vi "Measure DMM 3458A.vi"(8 "error in (no error)":errorcluster, 11 "VISA resource name":refnum<visa-resource-name>) -> (0 "error out":errorcluster, 3 "Display Value":sgl)   [LabVIEW 2016]
panel:
  out "Error Buffer":string
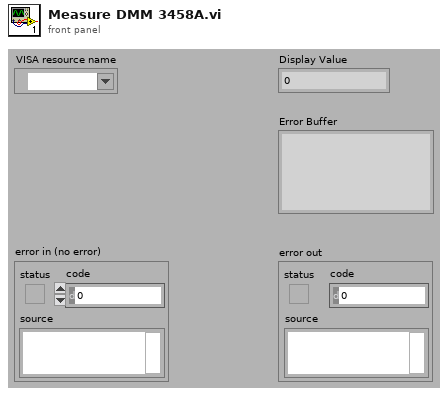
[diagram p1: front panel]
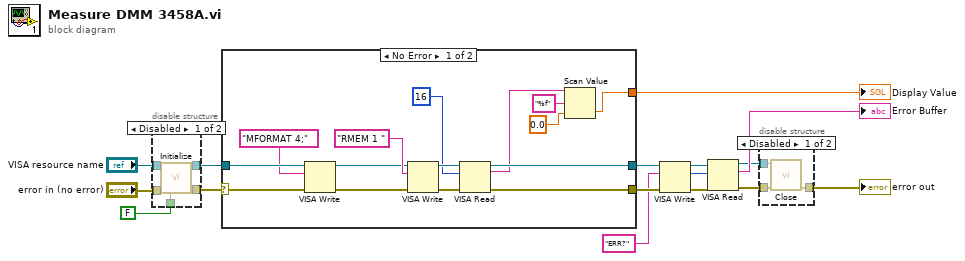
[diagram p0: block diagram]
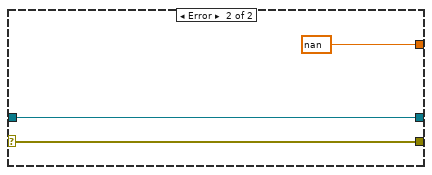
[diagram p4: hidden frame]
diagram:
  n1 = disable-structure shown="Disabled" {
    disable-tunnel: "error in (no error)" -> [w21 w22]
    disable-tunnel: [w20 w22] -> w7
    disable-tunnel: "VISA resource name" -> [w19 w23]
    disable-tunnel: [w18 w23] -> w5
    disable-tunnel: FALSE ("Reset?") -> [w17 _]
    frame Disabled {
      n2 = call <userlib>:"Initialize.vi"("error in (no error)"=w21, "Reset (True)"=w17, "VISA resource name"=w19) -> ("error out"=w20:errorcluster, "VISA resource name out"=w18:refnum<visa-resource-name>)  [unwired: 7 in]
    }
    frame Enabled {
    }
  }
  n3 = case shown="No Error" w7 {
    selector: w7 -> [w25 w41]
    tunnel: w5 -> [w33 w40]
    tunnel: [w34 w41] -> w16
    tunnel: [w35 w40] -> w15
    tunnel: [w24 sgl nan] -> w9
    frame No Error {
      n4 = VISA Write(VISA resource name=w33, write buffer="MFORMAT 4;", error in (no error)=w25) -> (VISA resource name out=w29:refnum<visa-resource-name>, error out=w28:errorcluster)  [unwired: 1 out]
      n5 = VISA Write(VISA resource name=w29, write buffer="RMEM 1 ", error in (no error)=w28) -> (VISA resource name out=w37:refnum<visa-resource-name>, error out=w38:errorcluster)  [unwired: 1 out]
      n6 = VISA Read(VISA resource name=w37, byte count=u32 16, error in (no error)=w38) -> (VISA resource name out=w35:refnum<visa-resource-name>, read buffer=w26:string, error out=w34:errorcluster)  [unwired: 1 out]
      n7 = Scan Value(string=w26, format string="%f", default (0 dbl)=sgl 0.0) -> (value=w24:sgl)  [unwired: 1 out]
    }
    frame Error {
    }
  }
  "Display Value" <- w9
  n8 = VISA Write(VISA resource name=w15, write buffer="ERR?", error in (no error)=w16) -> (VISA resource name out=w13:refnum<visa-resource-name>, return count=w12:u32, error out=w11:errorcluster)
  n9 = VISA Read(VISA resource name=w13, byte count=w12, error in (no error)=w11) -> (VISA resource name out=w2:refnum<visa-resource-name>, read buffer=→"Error Buffer":string, error out=w4:errorcluster)  [unwired: 1 out]
  n10 = disable-structure shown="Disabled" {
    disable-tunnel: w4 -> [w44 w45]
    disable-tunnel: [w43 w45] -> w3
    disable-tunnel: w2 -> [w42 _]
    frame Disabled {
      n11 = call <userlib>:"Close.vi"("error in (no error)"=w44, "VISA resource name"=w42) -> ("error out"=w43:errorcluster)  [unwired: 9 in]
    }
    frame Enabled {
    }
  }
  "error out" <- w3
